vi "Tosca-Create Flowchart From Template.vi"(0 "Name":string) -> (4 "Parameters out":refnum<class "Parameters.lvclass">, 6 "FSM out":refnum<class "FSM.Graph.lvclass">, 15 "error out":errorcluster)   [LabVIEW 2020]
uses:
  FSM Graph VIs/LV Source/Classes/FSM.Graph/FSM.Graph.lvclass
  Classes/Parameters/Parameters.lvclass
  Classes/Parameters/Parameters.lvclass/Parameters.ctl
  Classes/Parameters/Read Input Events.vi
  Classes/Parameters/Write Input Events.vi
  Tosca-Globals.vi
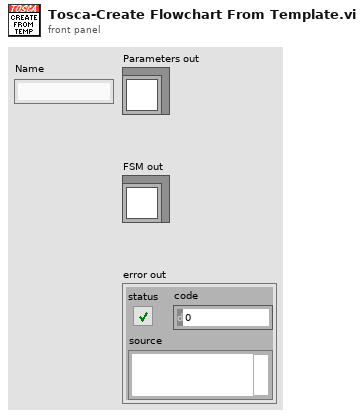
[diagram p1: front panel]
types:
  T1 = typedef "Tosca-Input Event.ctl" = cluster{"Name":string, "Criteria":T2[], "Operators":enum16{"AND", "OR"}[], "Accumulator":T4}
  T2 = typedef "Tosca-Input Criterion.ctl" = cluster{"DigInput":i32, "State":T3, "Time (ms)":i32, "Name":string}
  T3 = typedef "Logic State.ctl" = enum16{"Low", "High", "Rising", "Falling"}
  T4 = typedef "Tosca-Accumulator.ctl" = cluster{"active":bool, "N":i32, "T":dbl, "Imax":dbl, "latency":dbl}
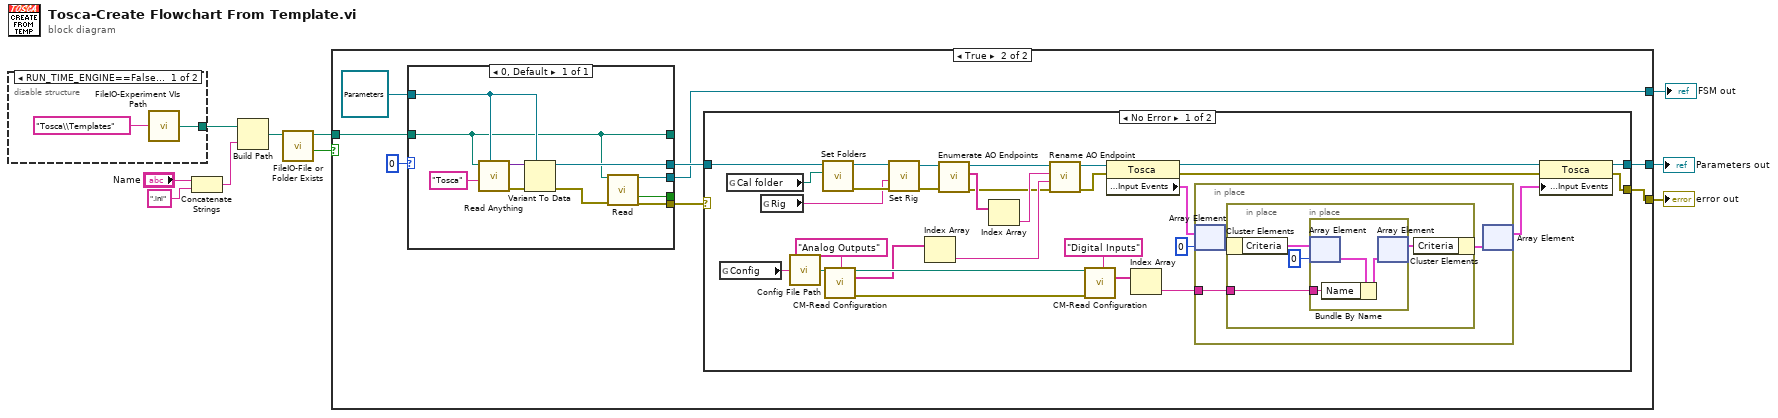
[diagram p0: block diagram]
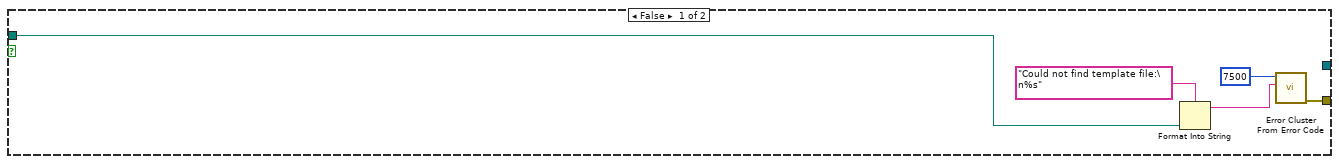
[diagram p2: hidden frame]
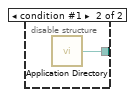
[diagram p4: hidden frame]
diagram:
  n1 = disable-structure shown="RUN_TIME_ENGINE==False, Default" {
    disable-tunnel: [w11 w13] -> w10
    frame condition #0 (active) {
      n2 = call "FileIO-Experiment VIs Path.vi"("relpath"="Tosca\\Templates") -> ("full path"=w11:path)  [unwired: 4 in]
    }
    frame condition #1 {
      n3 = call <vilib>:"Application Directory.vi"() -> ("Application Directory"=w13:path)
    }
  }
  n4 = Concatenate Strings("Name", ".ini" ("string")) -> (w5:string)
  n5 = Build Path(base path=w10, name or relative path=w5) -> (appended path=w3:path)
  n6 = call "FileIO-File or Folder Exists.vi"("path"=w3) -> ("Exists?"=w1:bool, "dup path"=w2:path)  [unwired: 7 in, 2 out]
  n7 = case shown="True" w1 {
    tunnel: w2 -> [w14 w25]
    tunnel: [_ w21] -> w8
    tunnel: [w18 w20] -> w7
    tunnel: [_ w19] -> w6
    frame False {
      n8 = Format Into String(format string="Could not find template file:\n%s", w14) -> (resulting string=w15:string)  [unwired: 2 in, 1 out]
      n9 = call <vilib>:"Error Cluster From Error Code.vi"("error message (\"\")"=w15, "error code (0)"=7500) -> ("error out"=w18:errorcluster)  [unwired: 7 in]
    }
    frame True {
      n10 = case shown="0, Default" 0 ("Version") {
        tunnel: [w72] -> w23
        tunnel: [w74] -> w22
        tunnel: w25 -> [w71]
        tunnel: [w71] -> _
        tunnel: refnum<class "Parameters.lvclass"> refnum ("Tosca") -> [w75]
        tunnel: [w70] -> _
        tunnel: [w69] -> w19
        frame 0, Default {
          n11 = call "Read Anything.vi"("Type of Anything"=w75, "Section Name (Name of \"Type of Anything\")"="Tosca" ("Section Name (Name of \"Anything\")"), "Path (dialog)"=w71) -> ("Error Out"=w77:errorcluster, "Anything"=w76:variant)  [unwired: 6 in, 1 out]
          n12 = Variant To Data(error in=w77, type=w75, Variant=w76) -> (data=w74:refnum<class "Parameters.lvclass">, error out=w73:errorcluster)
          n13 = call "Read.vi"("Path"=w71, "error in (no error)"=w73) -> ("FSM.Graph"=w69:refnum<class "FSM.Graph.lvclass">, "Success"=w70:bool, "error out"=w72:errorcluster)  [unwired: 11 in]
        }
      }
      n14 = case shown="No Error" w23 {
        selector: w23 -> [_ w67]
        tunnel: w22 -> [w56 w68]
        tunnel: [w53 w68] -> w21
        tunnel: [w52 w67] -> w20
        frame No Error {
          n15 = global read "Tosca-Globals.vi" "Config"() -> (w45:string)
          n16 = global read "Tosca-Globals.vi" "Cal folder"() -> (w49:path)
          n17 = global read "Tosca-Globals.vi" "Rig"() -> (w48:string)
          n18 = call "Config File Path.vi"("AppName"=w45) -> ("Default config file name"=w29:path)
          n19 = call "Set Folders.vi"("Calibration folder"=w49, "Tosca in"=w56) -> ("error out"=w50:errorcluster, "Tosca out"=w51:refnum<class "Parameters.lvclass">)  [unwired: 8 in]
          n20 = call "CM-Read Configuration.vi"("Connection File Path"=w29, "Section"="Analog Outputs") -> ("Connection File Path thru"=w31:path, "Names"=w27:string[], "error out"=w30:errorcluster)  [unwired: 9 in, 2 out]
          n21 = call "Set Rig.vi"("error in (no error)"=w50, "Rig"=w48, "Tosca in"=w51) -> ("error out"=w46:errorcluster, "Tosca out"=w47:refnum<class "Parameters.lvclass">)  [unwired: 7 in]
          n22 = Index Array(array=w27) -> (element=w41:string)  [unwired: 1 in]
          n23 = call "Enumerate AO Endpoints.vi"("error in (no error)"=w46, "Tosca in"=w47) -> ("error out"=w40:errorcluster, "Endpoints"=w44:string[], "Tosca out"=w43:refnum<class "Parameters.lvclass">)  [unwired: 7 in]
          n24 = Index Array(array=w44) -> (element=w42:string)  [unwired: 1 in]
          n25 = call "Rename AO Endpoint.vi"("error in (no error)"=w40, "New name"=w41, "Old name"=w42, "Tosca in"=w43) -> ("error out"=w38:errorcluster, "Tosca out"=w39:refnum<class "Parameters.lvclass">)  [unwired: 6 in]
          n26 = call "CM-Read Configuration.vi"("Connection File Path"=w31, "Section"="Digital Inputs", "error in (no error)"=w30) -> ("Names"=w28:string[])  [unwired: 8 in, 4 out]
          n27 = property class="Tosca"(reference=w39, error in=w38) -> (reference out=w55:refnum<class "Parameters.lvclass">, error out=w54:errorcluster, "Accessors:Input Events"=w35:T1[])
          n28 = Index Array(array=w28) -> (element=w36:string)  [unwired: 1 in]
          n29 = in-place {
            in-place-border: w36 -> [w58]
            n30 = in-place-array #1(w35, 0) -> (w59:T1)
            n31 = in-place {
              in-place-border: w58 -> [w62]
              n32 = in-place-cluster #2(w59) -> ("Criteria"=w61:T2[])
              n33 = in-place {
                in-place-border: w62 -> [w64]
                n34 = in-place-array #3(w61, 0) -> (w66:T2)
                n35 = Bundle By Name(cluster=w66, "Name"=w64) -> (w65:T2)
                n36 = in-place-array #3(w65) -> (w63:T2[])  [unwired: 1 out]
              }
              n37 = in-place-cluster #2("Criteria"=w63) -> (w57:T1)
            }
            n38 = in-place-array #1(w57) -> (w37:T1[])  [unwired: 1 out]
          }
          n39 = property class="Tosca"(reference=w55, error in=w54, "Accessors:Input Events"=w37) -> (reference out=w53:refnum<class "Parameters.lvclass">, error out=w52:errorcluster)
        }
        frame Error {
        }
      }
    }
  }
  "error out" <- w7
  "FSM out" <- w6
  "Parameters out" <- w8
